vi "coordinate.vi"() -> ()   [LabVIEW 2016]
uses:
  <vilib>/Analysis/NI_AALPro.lvlib
  <vilib>/Analysis/coordinate.llb/2D Cartesian Coordinate Shift (Scalar).vi
  <vilib>/Analysis/coordinate.llb/2D Cartesian Coordinate Rotation (Scalar).vi
panel:
  in  "theta":dbl
  out "appended array 2":dbl[](array[numeric])
  in  "IN array 2":dbl[](array[numeric])
  in  "shift":cluster{"dx":dbl, "dy":dbl}
  out "appended array":dbl[](array[numeric])
  in  "IN array":dbl[](array[numeric])
  out "x-y":dbl[](array[numeric])
  in  "Axis":dbl[](array[numeric])
  in  "origin":dbl[](array[numeric])
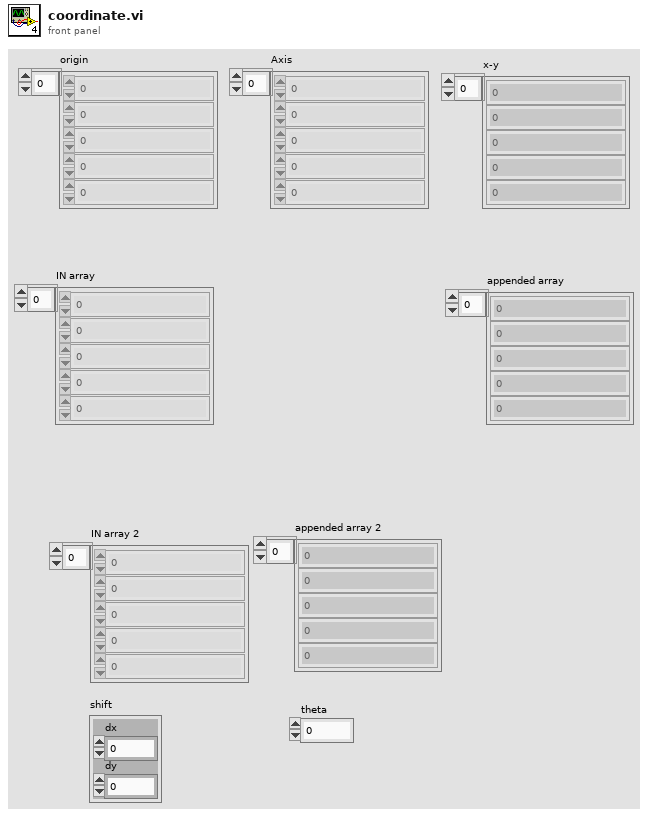
[diagram p1: front panel]
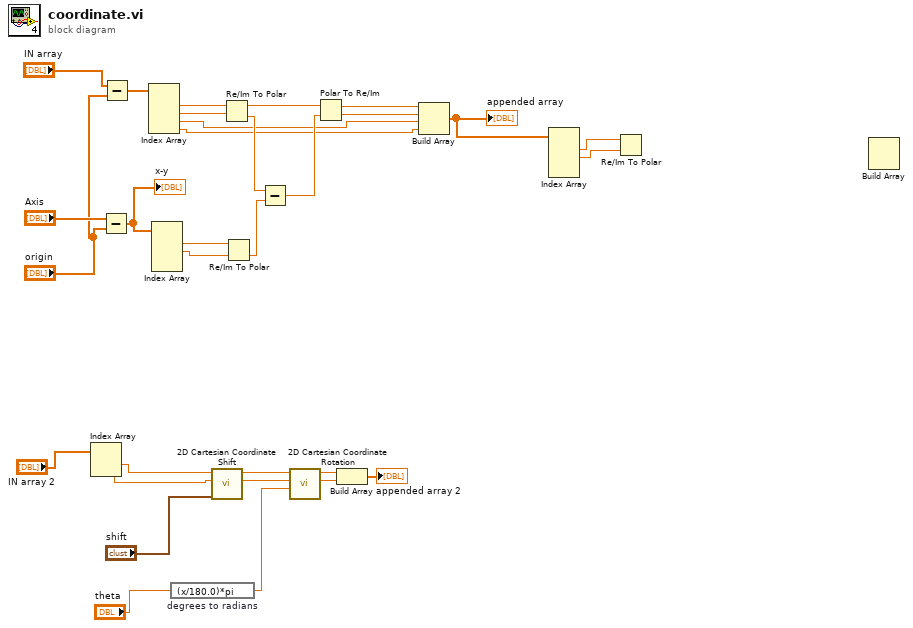
[diagram p0: block diagram]
diagram:
  n1 = Index Array(array="IN array 2") -> (element #1=w10:dbl, element #2=w9:dbl)  [unwired: 2 in]
  n2 = Subtract(x="Axis", y="origin") -> (x-y=w30:dbl[])
  "x-y" <- w30
  n3 = Subtract(x="IN array", y="origin") -> (x-y=w25:dbl[])
  n4 = Index Array(array=w25) -> (element #1=w24:dbl, element #2=w23:dbl, element #3=w16:dbl, element #4=w15:dbl)  [unwired: 4 in]
  n5 = Index Array(array=w30) -> (element #1=w29:dbl, element #2=w28:dbl)  [unwired: 4 in, 2 out]
  n6 = expression code="(x/180.0)*pi" "degrees to radians"("theta") -> (w5:dbl)
  n7 = call-poly <vilib>:"2D Cartesian Coordinate Shift.vi"("shift"="shift", "y"=w9, "x"=w10) -> ("y out"=w12:dbl, "x out"=w13:dbl)  [unwired: 6 in, 1 out]
  n8 = Re/Im To Polar(2:w23, 3:w24) -> (0:w22:dbl, 1:w19:dbl)
  n9 = Re/Im To Polar(2:w28, 3:w29) -> (0:w21:dbl)  [unwired: 1 out]
  n10 = Subtract(x=w22, y=w21) -> (x-y=w20:dbl)
  n11 = call-poly <vilib>:"2D Cartesian Coordinate Rotation.vi"("theta"=w5, "y"=w12, "x"=w13) -> ("y out"=w7:dbl, "x out"=w8:dbl)  [unwired: 6 in, 1 out]
  n12 = Polar To Re/Im(2:w20, 3:w19) -> (0:w17:dbl, 1:w18:dbl)
  n13 = Build Array(w8, w7) -> (→"appended array 2":dbl[])
  n14 = Build Array(w18, w17, w16, w15) -> (w3:dbl[])
  "appended array" <- w3
  n15 = Index Array(array=w3) -> (element #1=w2:dbl, element #2=w1:dbl)  [unwired: 4 in, 2 out]
  n16 = Re/Im To Polar(2:w1, 3:w2) -> ()  [unwired: 2 out]
  n17 = Build Array() -> ()  [unwired: 4 in, 1 out]
